vi "触摸屏绘画实验.vi"() -> ()   [LabVIEW 2011]
uses:
  <vilib>/STM32_DriverVI_Interface_F4/LCD/Brush Color_Index_F4.ctl
  <vilib>/eio/EIO_TerminalDirection.ctl
  <vilib>/STM32_DriverVI_Interface_F4/LCD/Show_Mode_F4.ctl
  <vilib>/STM32_DriverVI_Interface_F4/LCD/Font_Size_F4.ctl
  <vilib>/STM32_DriverVI_Interface_F4/LCD/LCD_Init_F4.vi
  <vilib>/STM32_DriverVI_Interface_F4/GPIO_EIO/GPI_EIO_Inner_F4.vi
  <vilib>/eio/EIONode/EIONode.xnode
panel:
  out "Init_success？":bool
  out "LCD_ID":u16 format="%x"
  in  "Brush Color":T1=enum."Red"
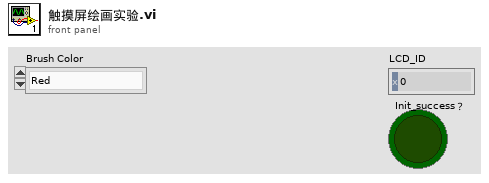
[diagram p1: front panel]
types:
  T1 = typedef "Brush Color_Index_F4.ctl" = enum8{"White", "Black", "Blue", "Green_Blue", "Red", "Magenta（品红）", "Green", "Cyan（青色）", "Yellow", "Brown", "Brown_Red", "Gray", "Dark_Blue", "Light_Blue", "Gray_Blue", "Light_Green", "Light_Gray", "Light_Gray_Blue", "Light_Brown_Blue"}
  T2 = enum8{"P0", "P1", "P2", "P3", "P4", "P5", "P6", "P7", "P8", "P9", "P10", "P11", "P12", "P13", "P14", "P15"}
  T3 = typedef "Show_Mode_F4.ctl" = enum8{"非叠加显示", "叠加显示"}
  T4 = typedef "Font_Size_F4.ctl" = enum8{"Small_Font（12）", "Big_Font（16）"}
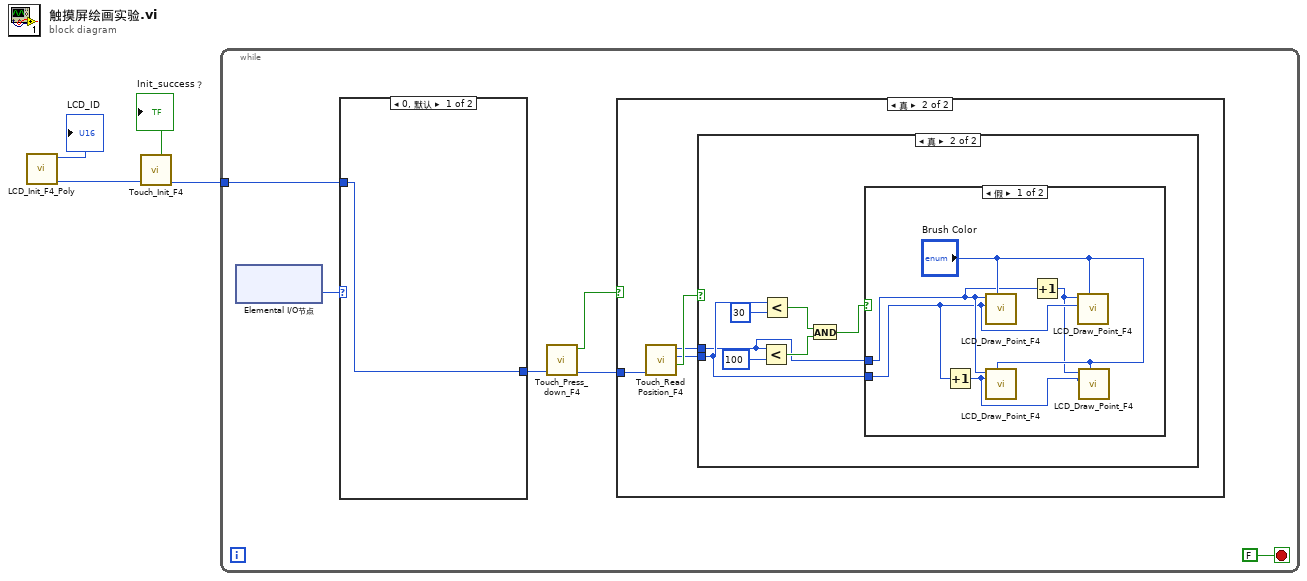
[diagram p0: block diagram]
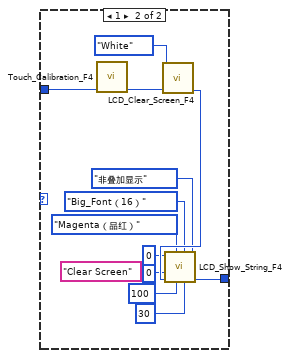
[diagram p5: hidden frame]
diagram:
  n1 = call-poly <vilib>:"LCD_Init_F4_Poly.vi"() -> ("err_out"=w4:u8, "LCD_ID"=→"LCD_ID":u16)  [unwired: 10 in]
  n2 = call <vilib>:"Touch_Init_F4.vi"("err_in"=w4) -> ("err_out"=w3:u8, "Init_success？"=→"Init_success？":bool)  [unwired: 9 in]
  n3 = while {
    tunnel: w3 -> [w10]
    stop <- FALSE stop-if-true
    n4 = xnode "Elemental I/O节点"() -> ("KEY_UP"=w9:u8)  [unwired: 1 in, 1 out]
    n5 = case shown="0, 默认" w9 {
      tunnel: w10 -> [w31 w44]
      tunnel: [w31 w33] -> w5
      frame 0, Default {
      }
      frame 1 {
        n6 = call <vilib>:"Touch_Calibration_F4.vi"("err_in"=w44) -> ("err_out"=w43:u8)  [unwired: 9 in, 1 out]
        n7 = call <vilib>:"LCD_Clear_Screen_F4.vi"("err_in"=w43, "Brush Color"=Brush_Color_Index_F4."White") -> ("err_out"=w42:u8)  [unwired: 9 in]
        n8 = call <vilib>:"LCD_Show_String_F4.vi"("Show_Mode"=Show_Mode_F4."非叠加显示", "Height"=u16 30, "Font_Size"=Font_Size_F4."Big_Font（16）", "Width"=u16 100, "Brush Color"=Brush_Color_Index_F4."Magenta（品红）", "err_in"=w42, "String"="Clear Screen", "Y_Position"=u16 0, "X_Position"=u16 0) -> ("err_out"=w33:u8)  [unwired: 2 in]
      }
    }
    n9 = call <vilib>:"Touch_Press_down_F4.vi"("err_in"=w5) -> ("err_out"=w8:u8, "Press_down？"=w7:bool)  [unwired: 9 in]
    n10 = case shown="真" w7 {
      tunnel: w8 -> [_ w14]
      frame False {
      }
      frame True {
        n11 = call <vilib>:"Touch_Read Position_F4.vi"("err_in"=w14) -> ("Read_valid?"=w13:bool, "Y_Position"=w11:u16, "X_Position"=w12:u16)  [unwired: 7 in, 1 out]
        n12 = case shown="真" w13 {
          tunnel: w12 -> [_ w15]
          tunnel: w11 -> [_ w16]
          frame False {
          }
          frame True {
            n13 = Less?(x=w15, y=u16 100) -> (x < y?=w18:bool)
            n14 = Less?(x=w16, y=u16 30) -> (x < y?=w19:bool)
            n15 = And(x=w19, y=w18) -> (x .and. y?=w17:bool)
            n16 = case shown="假" w17 {
              tunnel: w16 -> [w24 _]
              tunnel: w15 -> [w25 _]
              frame False {
                n17 = Increment(x=w24) -> (x+1=w22:u16)
                n18 = call <vilib>:"LCD_Draw_Point_F4.vi"("Brush Color"="Brush Color", "Y_Position"=w24, "X_Position"=w25) -> ()  [unwired: 8 in, 1 out]
                n19 = call <vilib>:"LCD_Draw_Point_F4.vi"("Brush Color"="Brush Color", "Y_Position"=w22, "X_Position"=w25) -> ()  [unwired: 8 in, 1 out]
                n20 = Increment(x=w25) -> (x+1=w23:u16)
                n21 = call <vilib>:"LCD_Draw_Point_F4.vi"("Brush Color"="Brush Color", "Y_Position"=w24, "X_Position"=w23) -> ()  [unwired: 8 in, 1 out]
                n22 = call <vilib>:"LCD_Draw_Point_F4.vi"("Brush Color"="Brush Color", "Y_Position"=w22, "X_Position"=w23) -> ()  [unwired: 8 in, 1 out]
              }
              frame True {
              }
            }
          }
        }
      }
    }
  }
